vi "BenchmarkIPBafe.vi"() -> ()   [LabVIEW 2017]
uses:
  <vilib>/Platform/TimedLoop/XDataNode/XDataNode.xnode
  <vilib>/Platform/TimedLoop/XDataNode/nitl_modes.ctl
  <vilib>/Platform/TimedLoop/XDataNode/XDNodeRunTimeDep.lvlib
  <vilib>/Platform/TimedLoop/XDataNode/wakeup.ctl
  <vilib>/Platform/TimedLoop/XDataNode/timing_clust.ctl
  AFE/Inputs.ctl
  AFE/ActiveFrontEnd.lvlib
  AFE/Gains.ctl
  AFE/Parameters.ctl
  AFE/Setpoint.ctl
  AFE/Range.ctl
  AFE/Signals.ctl
  AFE/ManualControl.ctl
  AFE/Actions.ctl
  AFE/Outputs.ctl
panel:
  out "A_timing":cluster{"ON":u32, "OFF":u32}
  out "feedback signals":cluster{"ready for input":bool}
  out "output valid 2":bool
  out "B_timing":cluster{"ON":u32, "OFF":u32}
  out "C_Timing":cluster{"ON":u32, "OFF":u32}
  out "Sector":u8
  in  "ref_alpha":sgl caption="voltage alpha"
  in  "input valid 2":bool=TRUE
  in  "ref_max":sgl=0.9999695
  in  "Period":i32=1
  in  "ref_beta":sgl caption="voltage beta"
  out "ready for input":bool
  out "output valid":bool
  out "AFE_Outputs":T1
  out "AFE_Actions":T2
  in  "AFE_ManualControl":T3
  in  "AFE_ControlSignals":T4
  in  "input valid":bool=TRUE
  in  "AFE_Ranges":T5={"PLL_PIRad_high"=inf, "PLL_PiRad_low"=inf, "IQcmd_high"=inf, "IQcmd_low"=inf, "IDcmd_high"=inf, "IDcmd_low"=inf, "VDcmd_high"=inf, "VDcmd_low"=inf, "VQmcd_high"=inf, "VQcmd_low"=inf}
  in  "AFE_Setpoints":T6
  in  "AFE_Params":T7
  in  "AFE_Gains":T8
  in  "AFE_Inputs":T9
  # "Device Utilization\n---------------------------\nTotal Slices: 51.7% (6875 out of 13300)\nSlice Registers: 16.1% (17155 out of 106400)\nSlice LUTs: 38.2% (20325 out of 53200)\nBlock RAMs: 21.4% (30 out of 140)\nDSP48s: 17.7% (39 out of 220)"
  # "Latency 153"
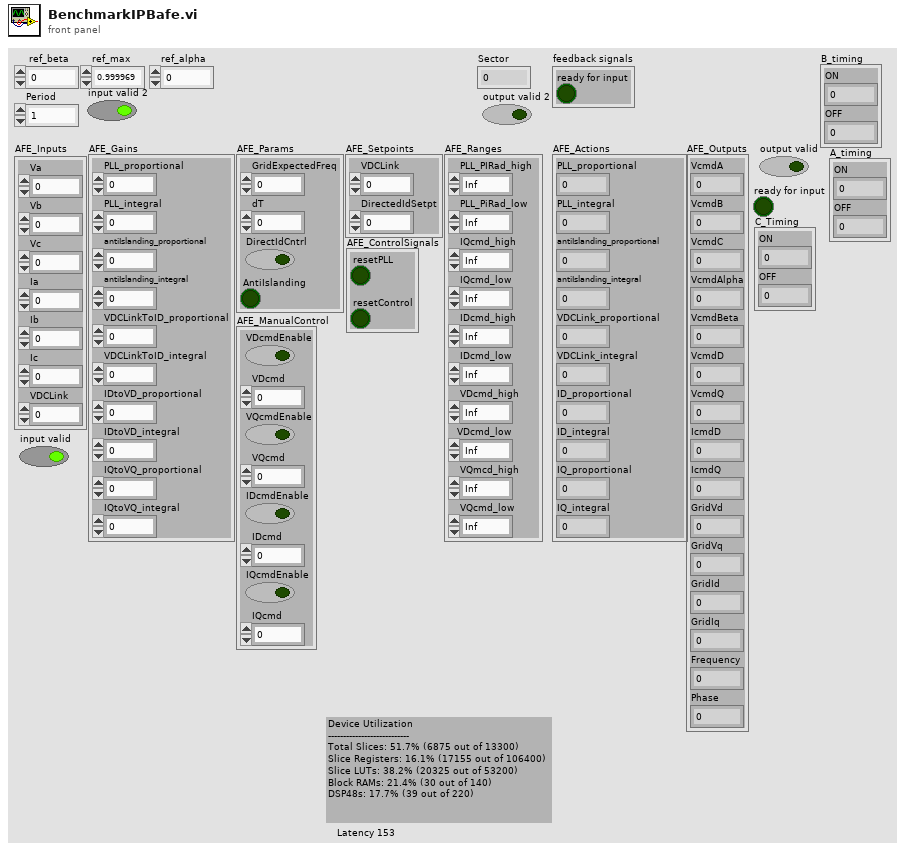
[diagram p1: front panel]
types:
  T1 = typedef "ActiveFrontEnd.lvlib/Outputs.ctl" = cluster{"VcmdA":sgl, "VcmdB":sgl, "VcmdC":sgl, "VcmdAlpha":sgl, "VcmdBeta":sgl, "VcmdD":sgl, "VcmdQ":sgl, "IcmdD":sgl, "IcmdQ":sgl, "GridVd":sgl, "GridVq":sgl, "GridId":sgl, "GridIq":sgl, "Frequency":sgl, "Phase":sgl}
  T2 = typedef "ActiveFrontEnd.lvlib/Actions.ctl" = cluster{"PLL_proportional":sgl, "PLL_integral":sgl, "antiIslanding_proportional":sgl, "antiIslanding_integral":sgl, "VDCLink_proportional":sgl, "VDCLink_integral":sgl, "ID_proportional":sgl, "ID_integral":sgl, "IQ_proportional":sgl, "IQ_integral":sgl}
  T3 = typedef "ActiveFrontEnd.lvlib/ManualControl.ctl" = cluster{"VDcmdEnable":bool, "VDcmd":sgl, "VQcmdEnable":bool, "VQcmd":sgl, "IDcmdEnable":bool, "IDcmd":sgl, "IQcmdEnable":bool, "IQcmd":sgl}
  T4 = typedef "ActiveFrontEnd.lvlib/Signals.ctl" = cluster{"resetPLL":bool, "resetControl":bool}
  T5 = typedef "ActiveFrontEnd.lvlib/Range.ctl" = cluster{"PLL_PIRad_high":sgl, "PLL_PiRad_low":sgl, "IQcmd_high":sgl, "IQcmd_low":sgl, "IDcmd_high":sgl, "IDcmd_low":sgl, "VDcmd_high":sgl, "VDcmd_low":sgl, "VQmcd_high":sgl, "VQcmd_low":sgl}
  T6 = typedef "ActiveFrontEnd.lvlib/Setpoint.ctl" = cluster{"VDCLink":sgl, "DirectedIdSetpt":sgl}
  T7 = typedef "ActiveFrontEnd.lvlib/Parameters.ctl" = cluster{"GridExpectedFreq":sgl, "dT":sgl, "DirectIdCntrl":bool, "AntiIslanding":bool}
  T8 = typedef "ActiveFrontEnd.lvlib/Gains.ctl" = cluster{"PLL_proportional":sgl, "PLL_integral":sgl, "antiIslanding_proportional":sgl, "antiIslanding_integral":sgl, "VDCLinkToID_proportional":sgl, "VDCLinkToID_integral":sgl, "IDtoVD_proportional":sgl, "IDtoVD_integral":sgl, "IQtoVQ_proportional":sgl, "IQtoVQ_integral":sgl}
  T9 = typedef "ActiveFrontEnd.lvlib/Inputs.ctl" = cluster{"Va":sgl, "Vb":sgl, "Vc":sgl, "Ia":sgl, "Ib":sgl, "Ic":sgl, "VDCLink":sgl}
  T10 = typedef "XDNodeRunTimeDep.lvlib/timing_clust.ctl" = cluster{"Expected End [f-1]":u64, "Actual End [f-1]":u64, "Finished Late? [f-1]":bool, "Expected End [i-1]":u64, "Actual End [i-1]":u64, "Finished Late? [i-1]":bool, "Expected Start [i]":u64, "Actual Start [i]":u64, "Expected Start [f]":u64, "Actual Start [f]":u64, "Source Name":string, "Structure Name":string, "Period":i64, "Deadline":i64, "Offset":i64, "Start":i64, "Priority":i32, "Timeout":i32, "Mode":T11, "Wakeup Reason":T12, "Error":errorcluster, "Source Type":string, "Secondary Source Type":string, "Global End Time":u64, "Global Start Time":u64, "Frame Duration":u64, "Iteration Duration":u64, "Assigned CPU":i32, "I/O Scan Engine Mode":u32}
  T11 = typedef "XDNodeRunTimeDep.lvlib/nitl_modes.ctl" = enum32{"No Change", "Process missed periods, maintain original phase", "Discard missed periods, maintain original phase", "Process missed periods, ignore original phase", "Discard missed periods, ignore original phase"}
  T12 = typedef "XDNodeRunTimeDep.lvlib/wakeup.ctl" = enum32{"Normal", "Aborted", "Asynchronous wakeup", "Timing source error", "Timed loop error", "Timeout"}
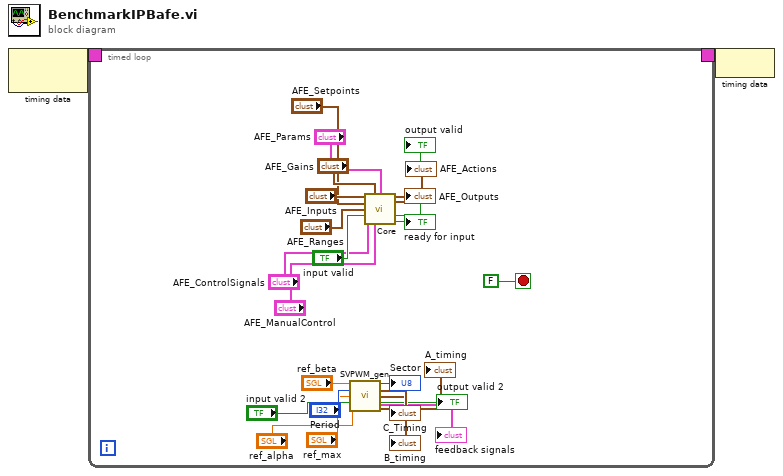
[diagram p0: block diagram]
diagram:
  n1 = node-c288() -> (w2:T10)  [unwired: 1 in]
  n2 = timed-loop {
    timing: w2 -> [_]
    timing-out: [_] -> w1
    stop <- FALSE stop-if-true
    n3 = call "SVPWM_gen.vi"("ref_beta"="ref_beta", "Period"="Period", "ref_max"="ref_max", "input valid"="input valid 2", "ref_alpha"="ref_alpha") -> ("Sector"=→"Sector":u8, "C_Timing"=→"C_Timing":cluster{"ON":u32, "OFF":u32}, "B_timing"=→"B_timing":cluster{"ON":u32, "OFF":u32}, "output valid"=→"output valid 2":bool, "feedback signals"=→"feedback signals":cluster{"ready for input":bool}, "A_timing"=→"A_timing":cluster{"ON":u32, "OFF":u32})  [unwired: 5 in]
    n4 = call "Core.vi"("AFE_Inputs"="AFE_Inputs", "AFE_Gains"="AFE_Gains", "AFE_Params"="AFE_Params", "AFE_Setpoints"="AFE_Setpoints", "AFE_Ranges"="AFE_Ranges", "input valid"="input valid", "AFE_ControlSignals"="AFE_ControlSignals", "AFE_ManualControl"="AFE_ManualControl") -> ("AFE_Actions"=→"AFE_Actions":T2, "AFE_Outputs"=→"AFE_Outputs":T1, "output valid"=→"output valid":bool, "ready for input"=→"ready for input":bool)  [unwired: 4 in]
  }
  n5 = node-c288(w1) -> ()
